vi "Notifier Send.vi"(8 "error in (no error)":errorcluster, 9 "Data":variant, 10 "Message":string, 11 "Messaging in":refnum<class "Messaging.lvclass">) -> (0 "error out":errorcluster, 3 "Messaging out":refnum<class "Messaging.lvclass">)   [LabVIEW 2023, in "Messaging.lvclass"]
uses:
  Messaging.lvclass
  Msg.Data.ctl
  Messaging.lvclass/Messaging.ctl
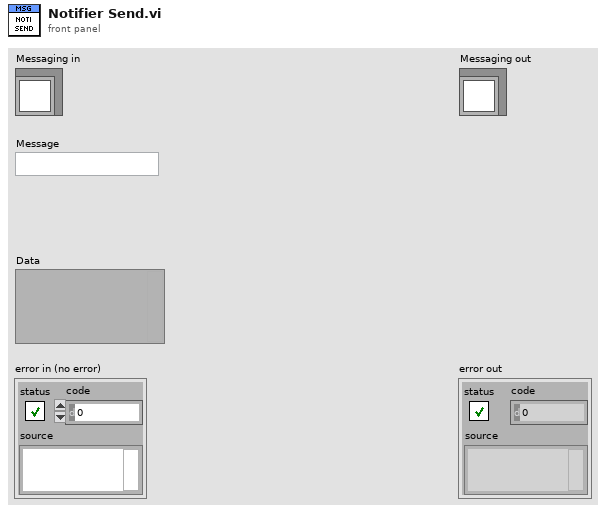
[diagram p1: front panel]
types:
  T1 = typedef "Messaging.lvclass/Msg.Data.ctl" = cluster{"Message":string, "Data":variant}
  T2 = typedef "Messaging.lvclass/Msg.Noti.Ref.ctl" = refnum<notifier>
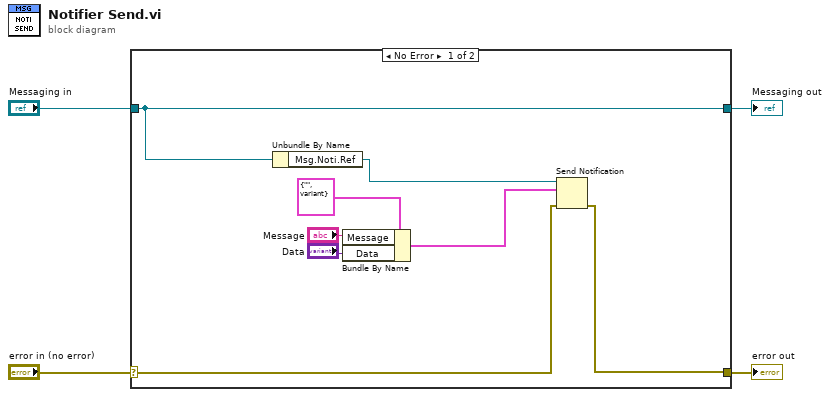
[diagram p0: block diagram]
diagram:
  n1 = case shown="No Error" "error in (no error)" {
    selector: "error in (no error)" -> [w5 w14]
    tunnel: [w6 w14] -> w3
    tunnel: [w7 w13] -> w1
    tunnel: "Messaging in" -> [w7 w13]
    frame No Error {
      n2 = Unbundle By Name(w7) -> ("Msg.Noti.Ref"=w8:T2)
      n3 = Bundle By Name(cluster=T1 {"Message"="", "Data"=variant} ("Msg.Q.Data"), "Message"="Message", "Data"="Data") -> (w9:T1)
      n4 = Send Notification(notification=w9, notifier=w8, error in (no error)=w5) -> (error out=w6:errorcluster)  [unwired: 1 out]
    }
    frame Error {
    }
  }
  "error out" <- w3
  "Messaging out" <- w1
